vi "AMWave.vi"() -> ()   [LabVIEW 2015]
uses:
  <vilib>/imath/engines/lvmath2/RunTimeEngine/Managers/WorkSpace/UID Generator.vi
  <vilib>/imath/engines/lvmath2/RunTimeEngine/RunTimeType/NIMS_RunTimeType_From StrictType (excl LVString).vi
  <instcachedir>/0/NIMS_RunTimeType_From StrictType (excl LVString)_EB1C38A9BC5048DA9ABDA8F781E54D21.lvgen/NIMS_RunTimeType_From StrictType (excl LVString)_EB1C38A9BC5048DA9ABDA8F781E54D21_000.vi
  <vilib>/imath/engines/lvmath2/RunTimeEngine/LocalVariableDefStatement/MC_LocalVariableDefStatement_Display.vi
  <vilib>/imath/engines/lvmath2/RunTimeEngine/RangeToken/NIMS_Range.vi
  <instcachedir>/0/NIMS_Range_D919CC09935940E88F755EC1C6F49AC1.lvgen/NIMS_Range_D919CC09935940E88F755EC1C6F49AC1_000.vi
  <vilib>/imathl/engines/lvmath/Functions/Error Handling/Create Error.vi
  <vilib>/imath/engines/lvmath2/RunTimeEngine/ArithmeticOperatorToken/NIMS_ArithmeticOperator_times.vi
  <instcachedir>/0/NIMS_ArithmeticOperator_times_DF26C4080E2A467BA28C929B8CF31953.lvgen/NIMS_ArithmeticOperator_times_DF26C4080E2A467BA28C929B8CF31953_000.vi
  <vilib>/imath/engines/lvmath2/RunTimeEngine/Managers/SymbolTable/Clear UID.vi
  <vilib>/imath/engines/lvmath2/RunTimeEngine/NodeEndStatement/NIMS_NodeEndStatement_Output.vi
  <instcachedir>/0/NIMS_NodeEndStatement_Output_53EC0D466D134D7ABD903AC30B43404B.lvgen/NIMS_NodeEndStatement_Output_53EC0D466D134D7ABD903AC30B43404B_005.vi
  <vilib>/imath/engines/lvmath2/RunTimeEngine/ErrorHandling/NIMS_Finalize Error.vi
  <vilib>/imath/engines/lvmath2/RunTimeEngine/Managers/SymbolTable/NIMS_WorkSpace.lvlib
panel:
  out "XY Graph":cluster{"t":dbl[], "x":dbl[]}(graph)
  out "AM Wave":cluster{"Time":dbl[], "Displacement":dbl[]}
  in  "AM Wave Properties":T1
  in  "Digitizing Parameters":T2
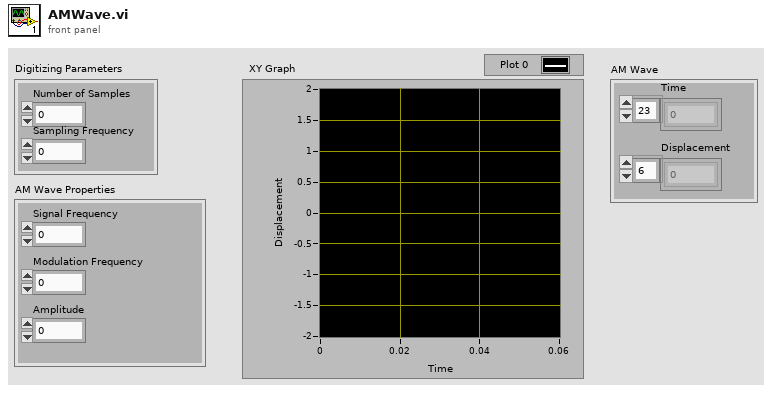
[diagram p1: front panel]
types:
  T1 = cluster{"Signal Frequency":dbl, "Modulation Frequency":dbl, "Amplitude":dbl}
  T2 = cluster{"Number of Samples":dbl, "Sampling Frequency":dbl}
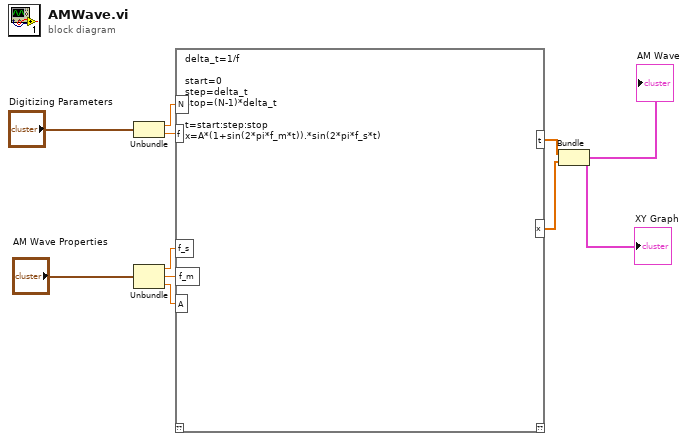
[diagram p0: block diagram]
diagram:
  n1 = Unbundle("Digitizing Parameters") -> ("Number of Samples"=w9:dbl, "Sampling Frequency"=w8:dbl)
  n2 = Unbundle("AM Wave Properties") -> ("Signal Frequency"=w6:dbl, "Modulation Frequency"=w5:dbl, "Amplitude"=w4:dbl)
  n3 = mathscript code="delta_t=1/f\n\nstart=0\nstep=delta_t\nstop=(N-1)*delta_t\n\nt=start:step:stop\nx=A*(1+sin(2*pi*f_m*t)).*sin(2*pi*f_s*t)"("f"=w8, "f_m"=w5, "A"=w4, "N"=w9, "f_s"=w6) -> ("t"=w3:dbl[], "x"=w2:dbl[])  [unwired: 1 in, 1 out]
  n4 = Bundle("t"=w3, "x"=w2) -> (→"AM Wave" →"XY Graph":cluster{"t":dbl[], "x":dbl[]})  [unwired: 1 in]
